vi "Cleanup.vi"(8 "error in (no error)":errorcluster, 11 "PathTreeNode in":refnum<class "PathTreeNode.lvclass">) -> (0 "error out":errorcluster)   [LabVIEW 2020, in "PathTree.lvlib" / "PathTreeNode.lvclass"]
uses:
  PathTreeNode.lvclass
  PathTreeNode.lvclass/PathTreeNode.ctl
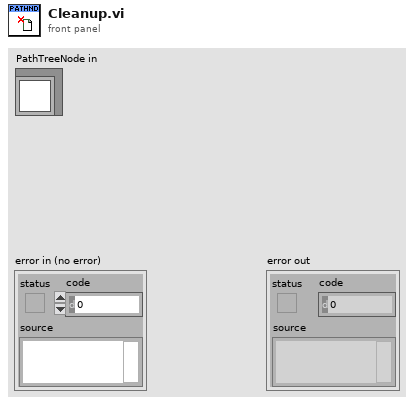
[diagram p1: front panel]
types:
  T1 = typedef "Advanced Structures.lvlib/PathTreeNode.lvclass/Ref Data.ctl" = cluster{"Tree":refnum<class>, "Parent":refnum<class>, "Token":string, "Child Tokens":string[], "Child Nodes":refnum<class>[], "Value":refnum<class>, "Has Value":bool}
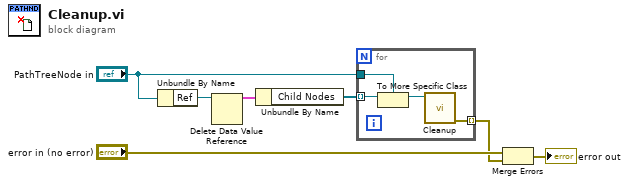
[diagram p0: block diagram]
diagram:
  n1 = Unbundle By Name("PathTreeNode in") -> ("Ref"=w6:refnum<data-value>)
  n2 = Delete Data Value Reference(data value reference=w6) -> (data value=w5:T1)  [unwired: 1 in, 1 out]
  n3 = Unbundle By Name(w5) -> ("Child Nodes"=w4:refnum<class>[])
  n4 = for {
    tunnel: w4 -> [w11] mode=indexing
    tunnel: "PathTreeNode in" -> [w10]
    tunnel: [w8] -> w1 mode=indexing
    n5 = To More Specific Class(target class=w10, reference=w11) -> (specific class reference=w9:refnum<class "PathTreeNode.lvclass">)  [unwired: 1 in, 1 out]
    n6 = call "Cleanup.vi"("PathTreeNode in"=w9) -> ("error out"=w8:errorcluster)  [unwired: 10 in]
  }
  n7 = Merge Errors("error in (no error)", w1) -> (→"error out":errorcluster)
